vi "DAQ_msgHandler Main.vi"() -> ()   [LabVIEW 2024]
doc: "This Continuous Measurement sample project is based on the Queued Message Handler template.\n\nThe Event Handling Loop generates messages based on user interface actions.\n\nThe Message Handling Loop processes messages generated by the Event Handling Loop, or by other messages. There are also Acquisition and Logging message handling loop subVIs, and a chart updating loop."
uses:
  Settings/Settings.ctl
  Acquisition/Hardware Configuration.ctl
  Acquisition/Signal Type.ctl
  Logging/Logging Configuration.ctl
  controls/DAQ_msgHandler UI State.ctl
  support/Message Queue/Enqueue Message (Single).vi
  <vilib>/Utility/error.llb/Error Cluster From Error Code.vi
  <vilib>/ErrorRing/Error Ring.xnode
  Acquisition/DAQ_msgHandler Acquisition.lvlib
  Settings/DAQ_msgHandler Settings.lvlib
  Logging/DAQ_msgHandler Logging.lvlib
  support/User Event - Stop/DAQ_msgHandler User Event - Stop.lvlib
  support/Message Queue/DAQ_msgHandler Message Queue.lvlib
  Settings/Settings Dialog.vi
panel:
  in  "Settings":bool
  in  "Start":bool
  in  "Stop":bool
  out "Status":string
  in  "Exit":bool
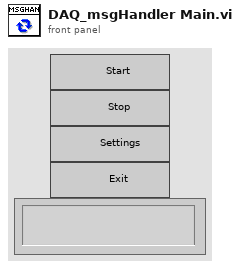
[diagram p1: front panel]
types:
  T1 = typedef "DAQ_msgHandler UI State.ctl" = enum16{"Idle", "Acquiring and Logging", "Waiting for Exit", "Waiting for Exit (Acq Stopped)", "Waiting for Exit (Log Stopped)", "Waiting for Stop", "Waiting for Stop (Acq Stopped)", "Waiting for Stop (Log Stopped)"}
  T2 = typedef "DAQ_msgHandler Settings.lvlib/Settings.ctl" = cluster{"Hardware Configuration":T3, "Logging Configuration":T5}
  T3 = typedef "DAQ_msgHandler Acquisition.lvlib/Hardware Configuration.ctl" = cluster{"HW Refnum <Replace Me>":string, "Signal Type <Replace Me>":T4}
  T4 = typedef "DAQ_msgHandler Acquisition.lvlib/Signal Type.ctl" = enum16{"Sine Wave", "Square with Noise"}
  T5 = typedef "DAQ_msgHandler Logging.lvlib/Logging Configuration.ctl" = cluster{"Log File Base Path":path, "TDMS File Reference":refnum<k34>}
  T6 = typedef "DAQ_msgHandler Message Queue.lvlib/All Message Queues.ctl" = cluster{"UI":refnum<queue>, "Acquisition":refnum<queue>, "Stream":refnum<queue>}
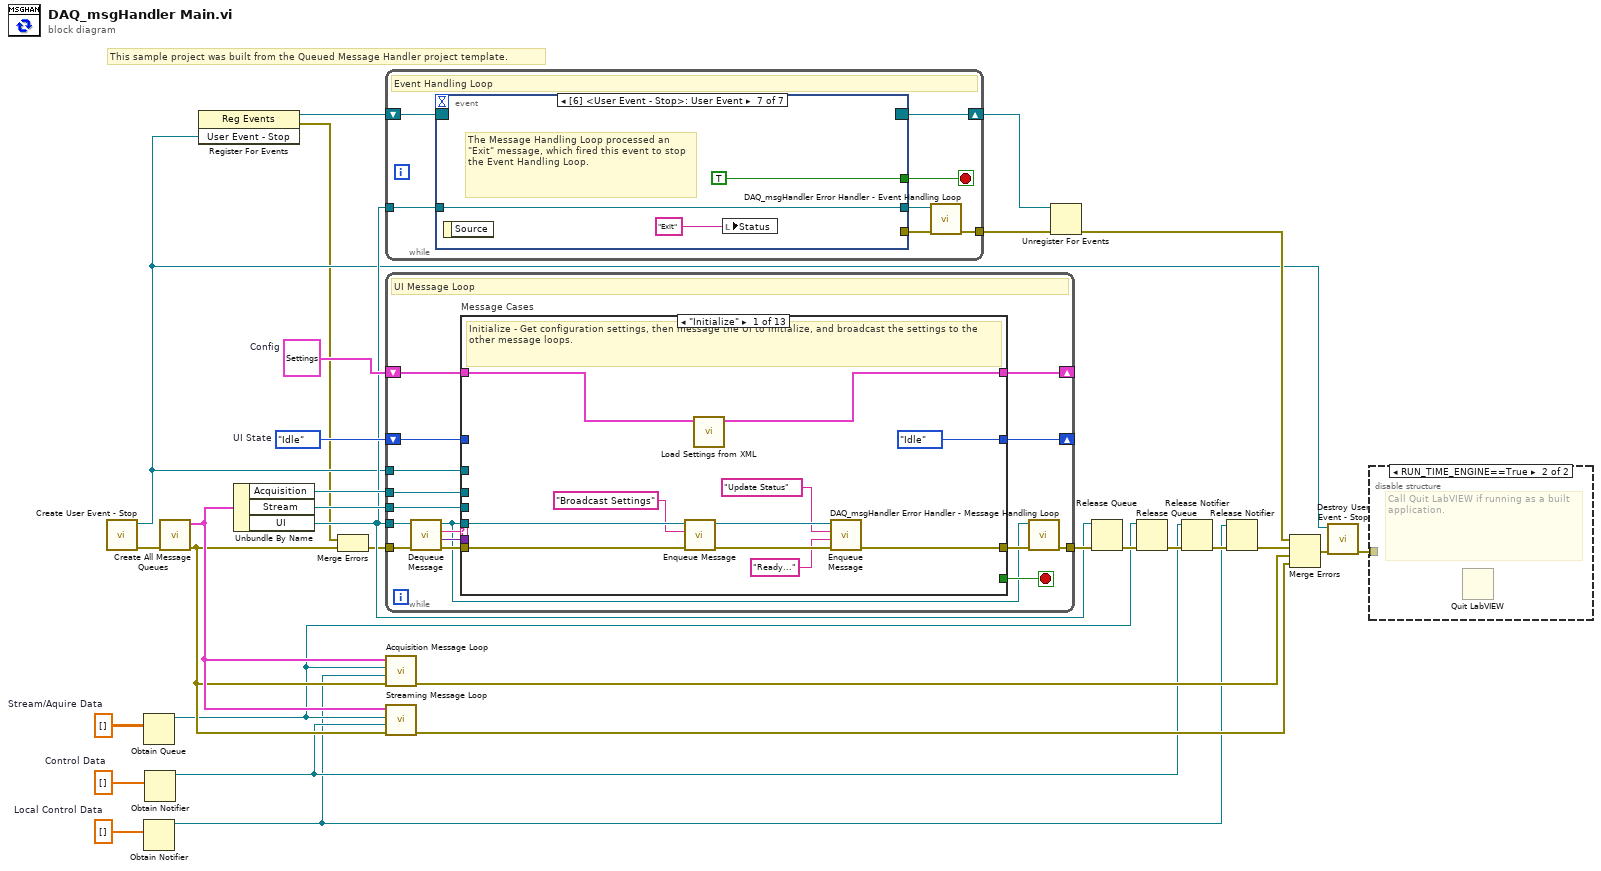
[diagram p0: block diagram]
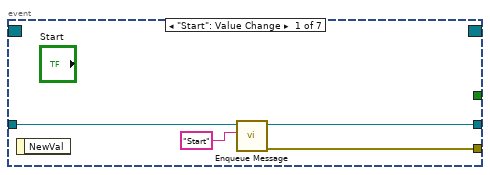
[diagram p3: hidden frame]
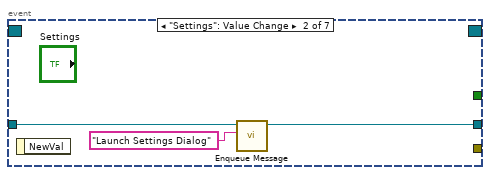
[diagram p4: hidden frame]
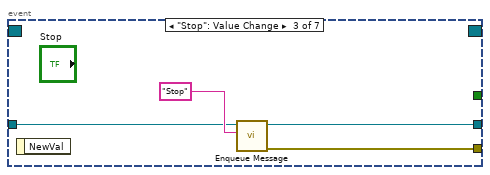
[diagram p5: hidden frame]
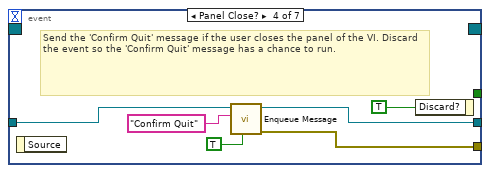
[diagram p6: hidden frame]
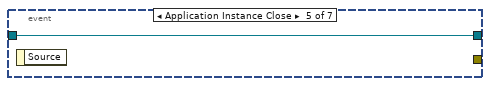
[diagram p7: hidden frame]
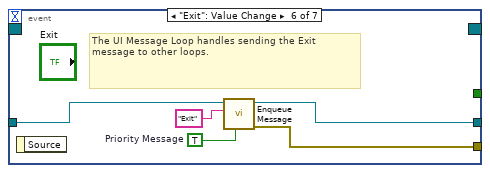
[diagram p8: hidden frame]
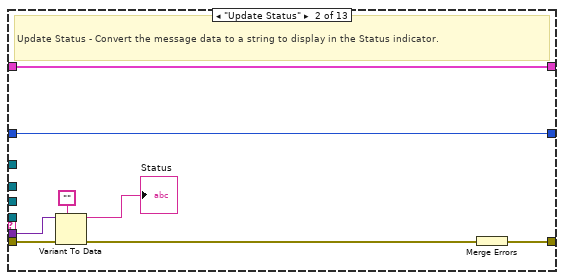
[diagram p9: hidden frame]
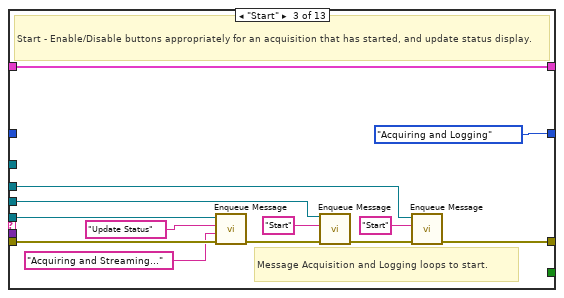
[diagram p10: hidden frame]
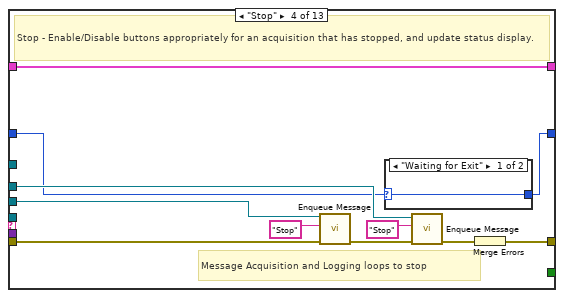
[diagram p11: hidden frame]
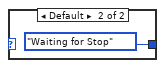
[diagram p12: hidden frame]
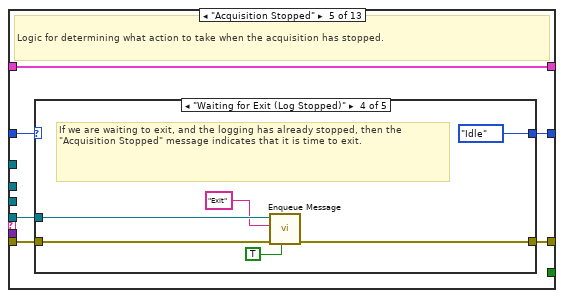
[diagram p13: hidden frame]
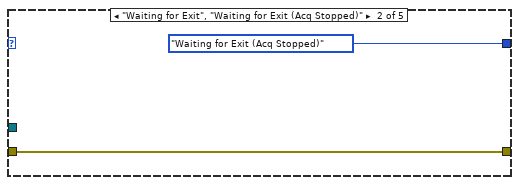
[diagram p15: hidden frame]
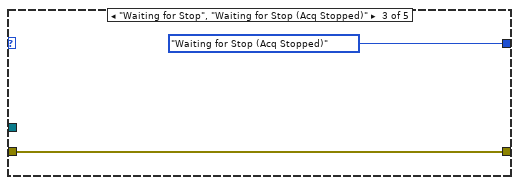
[diagram p16: hidden frame]
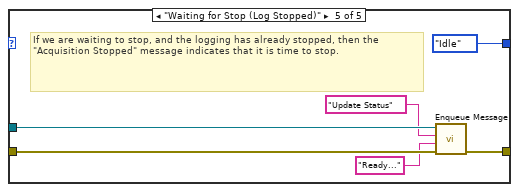
[diagram p17: hidden frame]
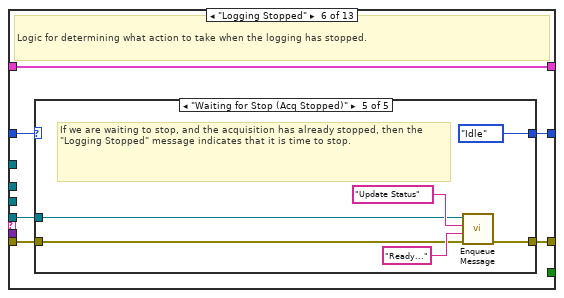
[diagram p18: hidden frame]
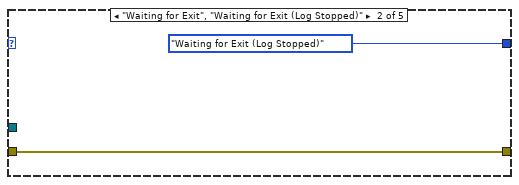
[diagram p20: hidden frame]
diagram:
  w2 = dbl[] []  # Local Control Data
  w6 = dbl[][] []  # Stream/Aquire Data
  w8 = dbl[] []  # Control Data
  w18 = DAQ_msgHandler_UI_State."Idle"  # UI State
  w23 = T2 {"Hardware Configuration"={"HW Refnum <Replace Me>"="", "Signal Type <Replace Me>"=enum."Sine Wave"}, "Logging Configuration"={"Log File Base Path"=path "", "TDMS File Reference"=refnum}}  # Config
  # "This sample project was built from the Queued Message Handler project template."
  n1 = call "Create User Event - Stop.vi"() -> ("error out"=w27:errorcluster, "User Event - Stop"=w11:refnum<user-event>)  [unwired: 10 in]
  n2 = Obtain Queue(element data type=w6) -> (queue out=w5:refnum<queue>)  [unwired: 4 in, 2 out]
  n3 = Obtain Notifier(notification data type=w2) -> (notifier out=w1:refnum<notifier>)  [unwired: 3 in, 2 out]
  n4 = Obtain Notifier(notification data type=w8) -> (notifier out=w7:refnum<notifier>)  [unwired: 3 in, 2 out]
  n5 = call "Create All Message Queues.vi"("error in (no error)"=w27) -> ("error out"=w24:errorcluster, "Message Queues out"=w26:T6)  [unwired: 9 in]
  n6 = register-events(w11) -> (reference out=w12:refnum<event-registration>, error out=w9:errorcluster)  [unwired: 2 in]
  n7 = Unbundle By Name(w26) -> ("Acquisition"=w20:refnum<queue>, "Stream"=w19:refnum<queue>, "UI"=w16:refnum<queue>)
  n8 = Merge Errors(w9, w24) -> (w10:errorcluster)
  n9 = while {
    tunnel: w16 -> [w36]
    tunnel: [w33] -> w29
    shift-right: [w35] -> w21
    shift-left: w12 -> [w37]
    stop <- w34 stop-if-true
    # "Event Handling Loop"
    n10 = event shown="[6] <User Event - Stop>: User Event" {
      selector: w37 -> [_ _ _ _ _ _ _]
      dyn-events: [_ _ _ _ _ _ _] -> w35
      timeout: _ -> [_ _ _ _ _ _ _]
      tunnel: [_ _ _ _ _ _ TRUE ("Discard?")] -> w34
      tunnel: w36 -> [w41 w43 w47 w52 w55 w57 w61]
      tunnel: [w39 _ w46 w50 _ w60 _] -> w32
      tunnel: [w38 w42 w45 w51 w55 w56 w61] -> w31
      event "Start": Value Change {
        n11 = event-data() -> ()  [unwired: 1 in, 1 out]
        n12 = call-poly "Enqueue Message.vi"("Message"="Start", "Message Queue"=w41) -> ("error out"=w39:errorcluster, "dup Message Queue"=w38:refnum<queue>)  [unwired: 8 in]
      }
      event "Settings": Value Change {
        n13 = event-data() -> ()  [unwired: 1 in, 1 out]
        n14 = call-poly "Enqueue Message.vi"("Message"="Launch Settings Dialog", "Message Queue"=w43) -> ("dup Message Queue"=w42:refnum<queue>)  [unwired: 8 in, 1 out]
      }
      event "Stop": Value Change {
        n15 = event-data() -> ()  [unwired: 1 in, 1 out]
        n16 = call-poly "Enqueue Message.vi"("Message"="Stop", "Message Queue"=w47) -> ("error out"=w46:errorcluster, "dup Message Queue"=w45:refnum<queue>)  [unwired: 8 in]
      }
      event Panel Close? {
        # "Send the 'Confirm Quit' message if the user closes the panel of the VI. Discard the event so the 'Confirm Quit' message has a chance to run."
        n17 = event-data() -> ()  [unwired: 1 in, 1 out]
        n18 = call-poly "Enqueue Message.vi"("Priority Message? (F)"=TRUE, "Message"="Confirm Quit", "Message Queue"=w52) -> ("error out"=w50:errorcluster, "dup Message Queue"=w51:refnum<queue>)  [unwired: 7 in]
        n19 = event-data("Discard?"=TRUE) -> ()  [unwired: 1 in, 1 out]
      }
      event Application Instance Close {
        n20 = event-data() -> ()  [unwired: 1 in, 1 out]
      }
      event "Exit": Value Change {
        w58 = TRUE  # Priority Message
        # "The UI Message Loop handles sending the Exit message to other loops."
        n21 = event-data() -> ()  [unwired: 1 in, 1 out]
        n22 = call-poly "Enqueue Message.vi"("Priority Message? (F)"=w58, "Message"="Exit", "Message Queue"=w57) -> ("error out"=w60:errorcluster, "dup Message Queue"=w56:refnum<queue>)  [unwired: 7 in]
      }
      event User Event {
        # "The Message Handling Loop processed an \"Exit\" message, which fired this event to stop the Event Handling Loop."
        n23 = event-data() -> ()  [unwired: 1 in, 1 out]
        n24 = local write "Status"("Exit" ("Exit String")) -> ()
      }
    }
    n25 = call "DAQ_msgHandler Error Handler - Event Handling Loop.vi"("error in (no error)"=w32, "Message Queue"=w31) -> ("dup error in"=w33:errorcluster)  [unwired: 8 in, 1 out]
  }
  n26 = while {
    tunnel: w16 -> [w73]
    tunnel: w11 -> [w78]
    shift-right: [w72] -> _
    shift-left: w23 -> [w71]
    tunnel: w20 -> [w70]
    tunnel: w19 -> [w69]
    shift-right: [w64] -> _
    shift-left: w18 -> [w65]
    tunnel: w10 -> [w77]
    tunnel: [w68] -> w30
    stop <- w79 stop-if-true
    # "UI Message Loop"
    n27 = call "Dequeue Message.vi"("error in (no error)"=w77, "Message Queue"=w73) -> ("error out"=w76:errorcluster, "Message Data"=w74:variant, "Message"=w75:string, "dup Message Queue"=w66:refnum<queue>)  [unwired: 6 in]
    n28 = case "Message Cases" shown="\"Initialize\"" w75 {
      selector: w75 -> [_ _ _ _ _ _ _ _ _ _ _ _ w252]
      tunnel: w66 -> [w83 _ w111 _ w127 w151 _ w188 _ w208 _ _ _]
      tunnel: w76 -> [w82 w97 w110 w121 w128 w152 w177 w190 w197 w207 w235 w250 _]
      tunnel: [w86 w98 w102 w122 w125 w149 w183 w184 w200 w206 w244 w249 w251] -> w67
      tunnel: [_ _ _ _ _ _ _ _ _ _ TRUE _ _] -> w79
      tunnel: w74 -> [_ w96 _ _ _ _ _ _ w201 _ w233 _ _]
      tunnel: w78 -> [_ _ _ _ _ _ _ _ _ _ w245 _ _]
      tunnel: [w89 w92 w109 w120 w130 w154 w181 w187 w204 w210 w243 w248 w254] -> w72
      tunnel: w71 -> [w90 w92 w109 w120 w130 w154 w181 w191 w204 w210 w243 w248 w254]
      tunnel: w70 -> [_ _ w101 w115 _ _ w175 _ _ _ w242 _ _]
      tunnel: w69 -> [_ _ w104 w118 _ _ w174 _ _ _ w241 _ _]
      tunnel: w65 -> [_ w91 _ w112 w129 w153 w173 w185 w199 w209 _ w247 w253]
      tunnel: [DAQ_msgHandler_UI_State."Idle" ("UI State") w91 DAQ_msgHandler_UI_State."Acquiring and Logging" ("UI State") w113 w126 w150 w173 w185 w199 w205 DAQ_msgHandler_UI_State."Idle" ("UI State") w247 w253] -> w64
      frame "Initialize" {
        # "Initialize - Get configuration settings, then message the UI to initialize, and broadcast the settings to the other message loops."
        n29 = call-poly "Enqueue Message.vi"("error in (no error)"=w82, "Message"="Broadcast Settings", "Message Queue"=w83) -> ("error out"=w88:errorcluster, "dup Message Queue"=w87:refnum<queue>)  [unwired: 7 in]
        n30 = call "Load Settings from XML.vi"("Settings in"=w90) -> ("Settings out"=w89:T2)  [unwired: 9 in, 1 out]
        n31 = call-poly "Enqueue Message.vi"("error in (no error)"=w88, "Message Data"="Ready..." ("Ready..."), "Message"="Update Status", "Message Queue"=w87) -> ("error out"=w86:errorcluster)  [unwired: 6 in, 1 out]
      }
      frame "Update Status" {
        # "Update Status - Convert the message data to a string to display in the Status indicator."
        n32 = Variant To Data(error in=w97, type="", Variant=w96) -> (data=→"Status":string, error out=w94:errorcluster)
        n33 = Merge Errors(w94) -> (w98:errorcluster)
      }
      frame "Start" {
        # "Message Acquisition and Logging loops to start."
        # "Start - Enable/Disable buttons appropriately for an acquisition that has started, and update status display."
        n34 = call-poly "Enqueue Message.vi"("error in (no error)"=w110, "Message Data"="Acquiring and Streaming..." ("Acquiring and Logging..."), "Message"="Update Status", "Message Queue"=w111) -> ("error out"=w106:errorcluster)  [unwired: 6 in, 1 out]
        n35 = call-poly "Enqueue Message.vi"("error in (no error)"=w106, "Message"="Start", "Message Queue"=w104) -> ("error out"=w103:errorcluster)  [unwired: 7 in, 1 out]
        n36 = call-poly "Enqueue Message.vi"("error in (no error)"=w103, "Message"="Start", "Message Queue"=w101) -> ("error out"=w102:errorcluster)  [unwired: 7 in, 1 out]
      }
      frame "Stop" {
        # "Message Acquisition and Logging loops to stop"
        # "Stop - Enable/Disable buttons appropriately for an acquisition that has stopped, and update status display."
        n37 = call-poly "Enqueue Message.vi"("error in (no error)"=w121, "Message"="Stop", "Message Queue"=w118) -> ("error out"=w117:errorcluster)  [unwired: 7 in, 1 out]
        n38 = case shown="\"Waiting for Exit\"" w112 {
          selector: w112 -> [w123 _]
          tunnel: [w123 DAQ_msgHandler_UI_State."Waiting for Stop" ("UI State")] -> w113
          frame "Waiting for Exit" {
          }
          frame Default {
          }
        }
        n39 = call-poly "Enqueue Message.vi"("error in (no error)"=w117, "Message"="Stop", "Message Queue"=w115) -> ("error out"=w116:errorcluster)  [unwired: 7 in, 1 out]
        n40 = Merge Errors(w116) -> (w122:errorcluster)
      }
      frame "Acquisition Stopped" {
        # "Logic for determining what action to take when the acquisition has stopped."
        n41 = case shown="\"Waiting for Exit (Log Stopped)\"" w129 {
          selector: w129 -> [w132 _ _ _ _]
          tunnel: w128 -> [w131 w134 w136 w142 w148]
          tunnel: w127 -> [_ _ _ w140 w145]
          tunnel: [w132 DAQ_msgHandler_UI_State."Waiting for Exit (Acq Stopped)" ("UI State") DAQ_msgHandler_UI_State."Waiting for Stop (Acq Stopped)" ("UI State") DAQ_msgHandler_UI_State."Idle" ("UI State") DAQ_msgHandler_UI_State."Idle" ("UI State")] -> w126
          tunnel: [w131 w134 w136 w141 w146] -> w125
          frame Default {
          }
          frame "Waiting for Exit", "Waiting for Exit (Acq Stopped)" {
          }
          frame "Waiting for Stop", "Waiting for Stop (Acq Stopped)" {
          }
          frame "Waiting for Exit (Log Stopped)" {
            # "If we are waiting to exit, and the logging has already stopped, then the \"Acquisition Stopped\" message indicates that it is time to exit."
            n42 = call-poly "Enqueue Message.vi"("Priority Message? (F)"=TRUE, "error in (no error)"=w142, "Message"="Exit", "Message Queue"=w140) -> ("error out"=w141:errorcluster)  [unwired: 6 in, 1 out]
          }
          frame "Waiting for Stop (Log Stopped)" {
            # "If we are waiting to stop, and the logging has already stopped, then the \"Acquisition Stopped\" message indicates that it is time to stop."
            n43 = call-poly "Enqueue Message.vi"("error in (no error)"=w148, "Message Data"="Ready..." ("Ready..."), "Message"="Update Status", "Message Queue"=w145) -> ("error out"=w146:errorcluster)  [unwired: 6 in, 1 out]
          }
        }
      }
      frame "Logging Stopped" {
        # "Logic for determining what action to take when the logging has stopped."
        n44 = case shown="\"Waiting for Stop (Acq Stopped)\"" w153 {
          selector: w153 -> [w156 _ _ _ _]
          tunnel: w152 -> [w155 w158 w160 w166 w169]
          tunnel: w151 -> [_ _ _ w164 w168]
          tunnel: [w156 DAQ_msgHandler_UI_State."Waiting for Exit (Log Stopped)" ("UI State") DAQ_msgHandler_UI_State."Waiting for Stop (Log Stopped)" ("UI State") DAQ_msgHandler_UI_State."Idle" ("UI State") DAQ_msgHandler_UI_State."Idle" ("UI State")] -> w150
          tunnel: [w155 w158 w160 w165 w167] -> w149
          frame Default {
          }
          frame "Waiting for Exit", "Waiting for Exit (Log Stopped)" {
          }
          frame "Waiting for Stop", "Waiting for Stop (Log Stopped)" {
          }
          frame "Waiting for Exit (Acq Stopped)" {
            # "If we are waiting to exit, and the acquisition has already stopped, then the \"Logging Stopped\" message indicates that it is time to exit."
            n45 = call-poly "Enqueue Message.vi"("Priority Message? (F)"=TRUE, "error in (no error)"=w166, "Message"="Exit", "Message Queue"=w164) -> ("error out"=w165:errorcluster)  [unwired: 6 in, 1 out]
          }
          frame "Waiting for Stop (Acq Stopped)" {
            # "If we are waiting to stop, and the acquisition has already stopped, then the \"Logging Stopped\" message indicates that it is time to stop."
            n46 = call-poly "Enqueue Message.vi"("error in (no error)"=w169, "Message Data"="Ready..." ("Ready..."), "Message"="Update Status", "Message Queue"=w168) -> ("error out"=w167:errorcluster)  [unwired: 6 in, 1 out]
          }
        }
      }
      frame "Broadcast settings" {
        w176 = "Update Settings" ("Message")
        # "Broadcast settings - Send the 'Update Settings' message to the Logging and Acquisition message loops."
        n47 = Unbundle By Name(w181) -> ("Hardware Configuration"=w180:T3, "Logging Configuration"=w179:T5)
        n48 = call-poly "Enqueue Message.vi"("Message Data"=w180, "Message"=w176, "Message Queue"=w175) -> ("error out"=w182:errorcluster)  [unwired: 7 in, 1 out]
        n49 = call-poly "Enqueue Message.vi"("error in (no error)"=w182, "Message Data"=w179, "Message"=w176, "Message Queue"=w174) -> ("error out"=w178:errorcluster)  [unwired: 6 in, 1 out]
        n50 = Merge Errors(w178, w177) -> (w183:errorcluster)
      }
      frame "Launch Settings Dialog" {
        # "Launch Settings Dialog - Launch the Settings Dialog when the user clicks the 'Settings' button."
        n51 = call-by-ref "?"("error in (no error)"=w190, "Settings in"=w191) -> ("error out"=w186:errorcluster, "Cancelled?"=w189:bool, "Settings out"=w187:T2)  [unwired: 8 in, 3 out]
        n52 = case shown="False" w189 {
          tunnel: w188 -> [w195 _]
          tunnel: w186 -> [w194 w196]
          tunnel: [w193 w196] -> w184
          frame False {
            n53 = call-poly "Enqueue Message.vi"("error in (no error)"=w194, "Message"="Broadcast Settings", "Message Queue"=w195) -> ("error out"=w193:errorcluster)  [unwired: 7 in, 1 out]
          }
          frame True {
          }
        }
      }
      frame "Error" {
        # "Error - Display an error dialog. This message is sent by the \"Error Handler\" VIs at the end of other loops in this application."
        n54 = Variant To Data(error in=w197, type=errorcluster {"status"=FALSE, "code"=0, "source"=""} ("error constant"), Variant=w201) -> (data=w198:errorcluster, error out=w202:errorcluster)
        n55 = call <vilib>:"Simple Error Handler.vi"("error in (no error)"=w198) -> ()  [unwired: 4 in, 5 out]
        n56 = Merge Errors(w202) -> (w200:errorcluster)
      }
      frame "Confirm Quit" {
        # "Confirm Quit - Message that can confirm whether or not the user wants to exit the application."
        n57 = case shown="\"Acquiring and Logging\"" w209 {
          tunnel: w208 -> [w216 w220]
          tunnel: w207 -> [w215 w219]
          tunnel: [w214 w218] -> w206
          tunnel: [DAQ_msgHandler_UI_State."Idle" ("UI State") w217] -> w205
          frame Default {
            # "If 'Confirm Quit' comes in while the system is idle, there is no need for a confirmation message."
            n58 = call-poly "Enqueue Message.vi"("Priority Message? (F)"=TRUE, "error in (no error)"=w215, "Message"="Exit", "Message Queue"=w216) -> ("error out"=w214:errorcluster)  [unwired: 6 in, 1 out]
          }
          frame "Acquiring and Logging" {
            n59 = Two Button Dialog(message="Are you sure you want to quit while the acquisition is running?" ("Confirm Quit Message"), 1:"No" ("No"), 2:"Yes" ("Yes")) -> (T button?=w221:bool)
            n60 = case shown="True" w221 {
              tunnel: w220 -> [_ w230]
              tunnel: w219 -> [w226 w231]
              tunnel: [w226 w229] -> w218
              tunnel: [DAQ_msgHandler_UI_State."Acquiring and Logging" ("UI State") DAQ_msgHandler_UI_State."Waiting for Exit" ("UI State")] -> w217
              frame False {
                # "User did not want to quit."
              }
              frame True {
                n61 = call-poly "Enqueue Message.vi"("error in (no error)"=w231, "Message"="Stop", "Message Queue"=w230) -> ("error out"=w229:errorcluster)  [unwired: 7 in, 1 out]
              }
            }
          }
        }
      }
      frame "Exit" {
        w237 = TRUE ("Priority Message? (F)")
        w238 = "Exit" ("Message")
        # "Popup an error dialog if 'Exit' was called as a result of an error."
        # "Stop the VI"
        # "Exit - Send Exit messages to the Acquisition and Logging loops, and fire the user event to stop the Event Handling Loop."
        n62 = Variant To Data(type=errorcluster {"status"=FALSE, "code"=0, "source"=""} ("error constant"), Variant=w233) -> (data=w232:errorcluster)  [unwired: 1 in, 1 out]
        n63 = call <vilib>:"Simple Error Handler.vi"("error in (no error)"=w232) -> ()  [unwired: 4 in, 5 out]
        n64 = call-poly "Enqueue Message.vi"("Priority Message? (F)"=w237, "error in (no error)"=w235, "Message"=w238, "Message Queue"=w242) -> ("error out"=w239:errorcluster)  [unwired: 6 in, 1 out]
        n65 = call-poly "Enqueue Message.vi"("Priority Message? (F)"=w237, "error in (no error)"=w239, "Message"=w238, "Message Queue"=w241) -> ("error out"=w236:errorcluster)  [unwired: 6 in, 1 out]
        n66 = call "Fire User Event - Stop.vi"("error in (no error)"=w236, "User Event - Stop"=w245) -> ("error out"=w244:errorcluster)  [unwired: 9 in]
      }
      frame "---Copy This Frame---" {
        # "Duplicate this frame when creating new messages.  Change this comment in the duplicated frame to describe this message."
        n67 = Merge Errors(w250) -> (w249:errorcluster)
      }
      frame Default {
        # "'Default' case only runs if there is a message that isn't defined in any of the other cases.  Output a programming error."
        n68 = xnode "Error Ring"("parameter 0"=w252) -> ("error out"=w251:errorcluster)
      }
    }
    n69 = call "DAQ_msgHandler Error Handler - Message Handling Loop.vi"("error in (no error)"=w67, "Message Queue"=w66) -> ("dup error in"=w68:errorcluster)  [unwired: 8 in, 1 out]
  }
  n70 = call "Acquisition Message Loop.vi"("error in (no error)"=w24, "local control"=w1, "queue out"=w5, "Message Queues"=w26) -> ("error out"=w28:errorcluster)  [unwired: 7 in]
  n71 = call "Streaming Message Loop.vi"("error in (no error)"=w24, "notifier out"=w7, "queue out"=w5, "Message Queues"=w26) -> ("error out"=w25:errorcluster)  [unwired: 7 in]
  n72 = Unregister For Events(event registration refnum=w21, error in=w29) -> (error out=w22:errorcluster)
  n73 = Release Queue(queue=w16, error in (no error)=w30) -> (error out=w14:errorcluster)  [unwired: 1 in, 2 out]
  n74 = Release Queue(queue=w5, error in (no error)=w14) -> (error out=w13:errorcluster)  [unwired: 1 in, 2 out]
  n75 = Release Notifier(notifier=w7, error in (no error)=w13) -> (error out=w4:errorcluster)  [unwired: 1 in, 2 out]
  n76 = Release Notifier(notifier=w1, error in (no error)=w4) -> (error out=w3:errorcluster)  [unwired: 1 in, 2 out]
  n77 = Merge Errors(w22, w3, w28, w25) -> (w17:errorcluster)
  n78 = call "Destroy User Event - Stop.vi"("error in (no error)"=w17, "User Event - Stop"=w11) -> ("error out"=w15:errorcluster)  [unwired: 9 in]
  n79 = disable-structure shown="RUN_TIME_ENGINE==True" {
    disable-tunnel: w15 -> [_ _]
    frame condition #0 (active) {
    }
    frame condition #1 {
      # "Call Quit LabVIEW if running as a built application."
      n80 = Quit LabVIEW() -> ()  [unwired: 1 in]
    }
  }
